vi "Draw.vi"(0 "FSM.Label":refnum<class "FSM.Label.lvclass">, 7 "picture in":picture, 11 "selected":bool) -> (4 "FSM.Label thru":refnum<class "FSM.Label.lvclass">, 8 "picture out":picture)   [LabVIEW 2020, in "FSM.Label.lvclass"]
uses:
  FSM.Label.lvclass
  FSM.Label.lvclass/FSM.Label.ctl
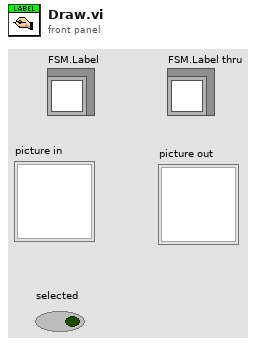
[diagram p1: front panel]
types:
  T1 = cluster{"left":i16, "top":i16, "right":i16, "bottom":i16}
  T2 = cluster{"Font Name:":string, "Size":i16, "Strikeout?":bool, "Italic?":bool, "Underline?":bool, "Outline?":bool, "Shadow?":bool, "Bold?":bool}
  T3 = cluster{"horizontal":enum16{"left", "center", "right"}, "vertical":enum16{"top", "center", "bottom"}}
  T4 = cluster{"Width":i16, "Style":enum32{"Solid", "Dash", "Dot", "DashDot", "DashDotDot"}}
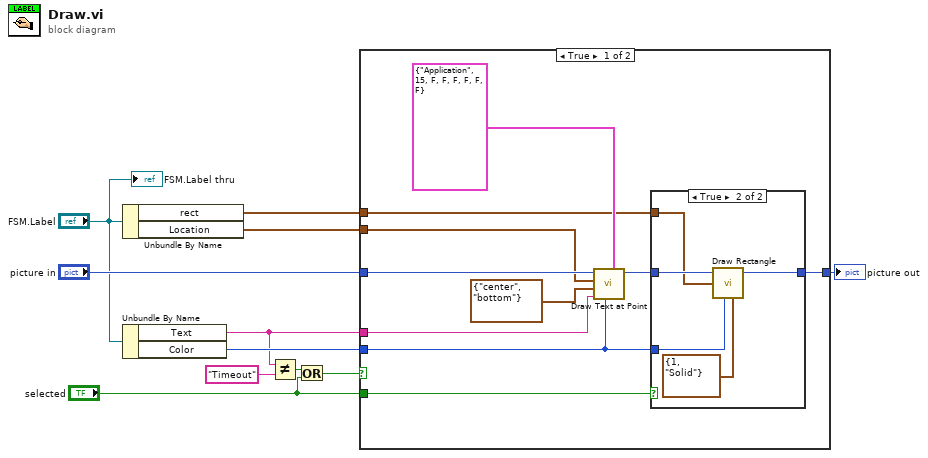
[diagram p0: block diagram]
diagram:
  n1 = Unbundle By Name("FSM.Label") -> ("rect"=w6:T1, "Location"=w10:cluster{"x":i16, "y":i16})
  n2 = Unbundle By Name("FSM.Label") -> ("Text"=w5:string, "Color"=w7:u32)
  n3 = Not Equal?(x=w5, y="Timeout") -> (x != y?=w3:bool)
  n4 = Or(x=w3, y="selected") -> (x .or. y?=w1:bool)
  n5 = case shown="True" w1 {
    tunnel: "picture in" -> [w21 w28]
    tunnel: w10 -> [w20 _]
    tunnel: "selected" -> [w16 _]
    tunnel: [w14 w28] -> w8
    tunnel: w7 -> [w13 _]
    tunnel: w6 -> [w12 _]
    tunnel: w5 -> [w18 _]
    frame True {
      n6 = call <vilib>:"Draw Text at Point.vi"("[user-specified font]"=T2 {"Font Name:"="Application", "Size"=15, "Strikeout?"=FALSE, "Italic?"=FALSE, "Underline?"=FALSE, "Outline?"=FALSE, "Shadow?"=FALSE, "Bold?"=FALSE}, "text color(black)"=w13, "text"=w18, "alignment(left, top)"=T3 {"horizontal"=enum."center", "vertical"=enum."bottom"}, "origin"=w20, "picture"=w21) -> ("new picture"=w15:picture)  [unwired: 4 in, 1 out]
      n7 = case shown="True" w16 {
        tunnel: w15 -> [w22 w27]
        tunnel: [w22 w26] -> w14
        tunnel: w13 -> [_ w25]
        tunnel: w12 -> [_ w23]
        frame False {
        }
        frame True {
          n8 = call <vilib>:"Draw Rectangle.vi"("picture"=w27, "rect"=w23, "color(black)"=w25, "pen"=T4 {"Width"=1, "Style"=enum."Solid"}) -> ("new picture"=w26:picture)  [unwired: 5 in]
        }
      }
    }
    frame False {
    }
  }
  "picture out" <- w8
  "FSM.Label thru" <- "FSM.Label"
